vi "CRYConvert ASCII to Unicode.vi"(4 "ASCII":string, 5 "Code Page":u32(ring) items=["System default"=0, "Latin-1"=1252, "Japanese"=932, "Korean"=949, "Chinese simplified"=936, "Chinese traditional"=950, "Central Europe"=1250, "Cyrillic"=1251, "Greek"=1253, "Turkish"=1254, "Hebrew"=1255, "Arabic"=1256, "Baltic"=1257, "Thai"=874, "Vietnamese"=783, "UTF8"=65001, "UTF-7"=65000]) -> (1 "Unicode":string)   [LabVIEW 2013]
uses:
  Kernel32.DLL
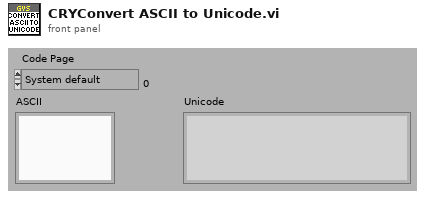
[diagram p1: front panel]
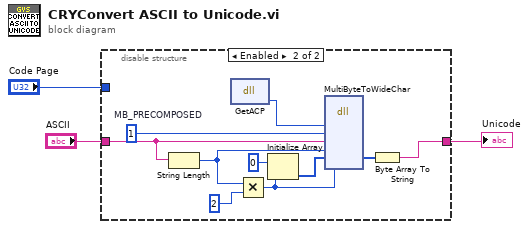
[diagram p0: block diagram]
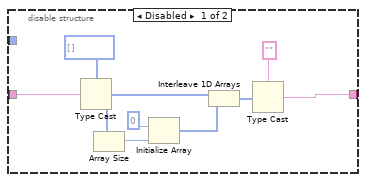
[diagram p2: hidden frame]
diagram:
  n1 = disable-structure shown="Enabled" {
    disable-tunnel: "ASCII" -> [w12 w16]
    disable-tunnel: [w4 w15] -> w2
    disable-tunnel: "Code Page" -> [_ _]
    frame Disabled {
      n2 = Type Cast(type=u8[] [], x=w12) -> (*(type *) &x=w8:u8[])
      n3 = Array Size(array=w8) -> (size(s)=w10:i32)
      n4 = Initialize Array(u8 0, w10) -> (w7:u8[])
      n5 = Interleave 1D Arrays(w8, w7) -> (w6:u8[])
      n6 = Type Cast(type="", x=w6) -> (*(type *) &x=w4:string)
    }
    frame Enabled {
      w21 = u32 1  # MB_PRECOMPOSED
      n7 = String Length(string=w16) -> (length=w14:i32)
      n8 = dll-call lib="kernel32.dll" fn="GetACP" label="GetACP()"() -> (w13:u32)  [unwired: 3 in, 2 out]
      n9 = Multiply(x=w14, y=2) -> (x*y=w17:i32)
      n10 = Initialize Array(u8 0, w17) -> (w19:u8[])
      n11 = dll-call lib="kernel32.dll" fn="MultiByteToWideChar"("codePage"=w13, "dwFlags"=w21, "pMultiByteStr"=w16, "cbMultiByte"=w14, "lpWideCharStr"=w19, "cchWideChar"=w17) -> ("lpWideCharStr"=w18:u8[])  [unwired: 8 in, 3 out]
      n12 = Byte Array To String(unsigned byte array=w18) -> (string=w15:string)
    }
  }
  "Unicode" <- w2
